vi "Update Chnls SyncHW.vi"(8 "error in (no error)":errorcluster, 10 "ChnlSettings":T1[](array[typedef]) {"ChnParameter"."Delay (µs)" min=0.0 max=100000000.0 format="%.4f"; "G08_Chnl_Settings"."Pulse Width (µs)" min=0.0 max=8947840.0 format="%#.6f"; "Go and Done Signal"."Done Signal" format="%04x" items=["Local Primary"=1, "Local Secondary"=2, "Local Force"=4, "Master Primary"=16]; "Go and Done Signal"."Go Signal" format="%04x" items=["Local Primary0x1"=1, "Local Secondary0x2"=2, "Local Force 0x4"=4, "Resynchronize 0x8"=8, "Master Prim. 0x10"=16, "Master Sec. 0x20"=32, "Master Force  0x40"=64, "System Clock 0x80"=128, "Delay Clock 0x100"=256, "Inhibit Local 0x200"=512, "Start Local 0x400"=1024, "Start Bus 0x800"=2048, "Step Back Local 0x1000"=4096, "Step Back Bus 0x2000"=8192, "RunCircle 0x4000"=16384, "SyncReload 0x8000"=32768, "From E 0x10000"=65536, "From F 0x20000"=131072, "From Bus 0x40000"=262144]}, 11 "BME_DG_System in":refnum<class "BME_DG_System.lvclass">) -> (0 "error out":errorcluster, 2 "ProblemChnls":string[](array[string]), 3 "BME_DG_System out":refnum<class "BME_DG_System.lvclass">)   [LabVIEW 2009, in "POLARIS BME DG.lvlib" / "BME_DG_System.lvclass"]
doc: "VI works with SG08P2 based systems. SG08P2 store new parameter in a buffer and waits for appropriate moment to activate they.\n\nFirst VI check the integrity of new chnl settints. Then it writes settings in channel objects. Last it uptates HW and call DLL SyncLoadAllCard. This allows the card to change to new parameters at next common output modulo counter. \n\n\n---------------\n\nauthor: Alexander Kessler, Helmholtz-Institut-Jena \nmaintainer: Alexander Kessler: alexander.kessler@uni-jena.de\n\n\nLicense Agreement for this software:\n\nCopyright (C)\nHelmholtz-Institut-Jena\nFröbelsteg 3\n07743 Jena\nGermany\n\nContact: alexander.kessler@uni-jena.de\n\nThis program is free software; you can redistribute it and/or modify it under the terms of the GNU General Public License as published by the Free Software Foundation; either version 2 of the license, or (at your option) any later version.\n\nThis program is distributed in the hope that it will be useful, but WITHOUT ANY WARRANTY; without even the implied warranty of MERCHANTABILITY or FITNESS FOR A PARTICULAR PURPOSE. See the GNU General License for more details (http://www.gnu.org)."
uses:
  BME_DG_System.lvclass
  LV-BME Interface/Chnl Settings Complete.ctl
  LV-BME Interface/ChnlSettings.ctl
  LV-BME Interface/Go_Done_Chnl_Settings.ctl
  LV-BME Interface/GoSignalBits.ctl
  LV-BME Interface/SG08_Chnl_Settings.ctl
  BME_DG_Chnl/BME_DG_Chnl.lvclass
  POLARIS BME DG.lvlib
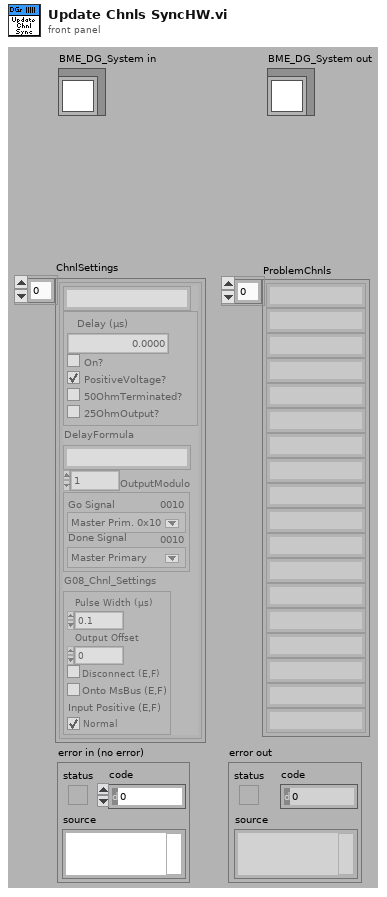
[diagram p1: front panel]
types:
  T1 = typedef "POLARIS BME DG.lvlib/Chnl Settings Complete.ctl" = cluster{"Channel Name":string, "ChnParameter":T2, "DelayFormula":string, "OutputModulo":i32, "Go and Done Signal":T3, "G08_Chnl_Settings":T5}
  T2 = typedef "POLARIS BME DG.lvlib/ChnlSettings.ctl" = cluster{" Delay (µs)":dbl, "On?":bool, "PositiveVoltage?":bool, "50OhmTerminated? ":bool, "25OhmOutput?":bool}
  T3 = typedef "POLARIS BME DG.lvlib/Go_Done_Chnl_Settings.ctl" = cluster{"Go Signal":T4, "Done Signal":u32}
  T4 = typedef "POLARIS BME DG.lvlib/GoSignalBits.ctl" = u32
  T5 = typedef "POLARIS BME DG.lvlib/SG08_Chnl_Settings.ctl" = cluster{"Pulse Width (µs)":dbl, "Output Offset":u32, "Disconnect (E,F)":bool, "Onto MsBus (E,F)":bool, "Input Positive (E,F)":bool}
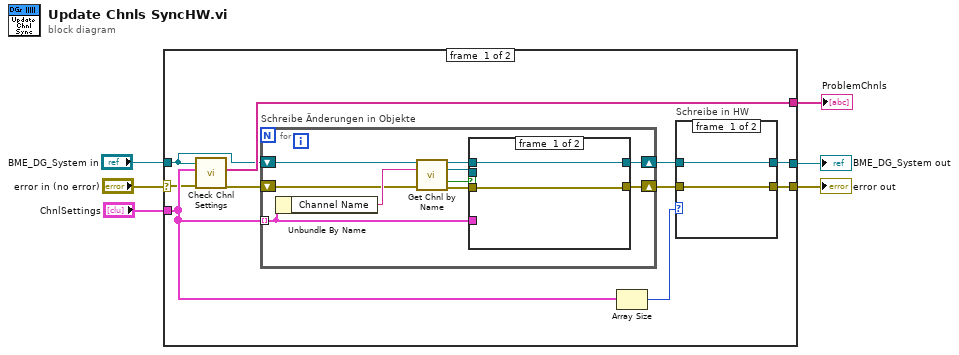
[diagram p0: block diagram]
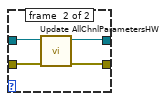
[diagram p2: hidden frame]
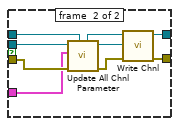
[diagram p3: hidden frame]
diagram:
  n1 = case shown="No Error" "error in (no error)" {
    selector: "error in (no error)" -> [w10 w45]
    tunnel: [w12 w45] -> w6
    tunnel: [w13 w44] -> w5
    tunnel: "BME_DG_System in" -> [w7 w44]
    tunnel: "ChnlSettings" -> [w11 _]
    tunnel: [w9 _] -> w1
    frame #0 {
      n2 = call "Check Chnl Settings.vi"("error in (no error)"=w10, "ChnlSettings"=w11, "BME_DG_System in"=w7) -> ("error out"=w8:errorcluster, "Problem Chnls out"=w9:string[])  [unwired: 7 in]
      n3 = for "Schreibe Änderungen in Objekte" {
        shift-right: [w27] -> w15
        shift-left: w7 -> [w28]
        tunnel: w11 -> [w23] mode=indexing
        shift-right: [w24] -> w14
        shift-left: w8 -> [w25]
        n4 = Unbundle By Name(w23) -> ("Channel Name"=w26:string)
        n5 = call "Get Chnl by Name.vi"("BME_DG_System in"=w28, "Chnl Name"=w26, "error in (no error)"=w25) -> ("BME_DG_System out"=w30:refnum<class "BME_DG_System.lvclass">, "BME_DG_Chnl"=w31:refnum<class "BME_DG_Chnl.lvclass">, "found?"=w32:bool, "error out"=w29:errorcluster)  [unwired: 7 in, 2 out]
        n6 = case shown="True" w32 {
          tunnel: w31 -> [_ w40]
          tunnel: w30 -> [w34 w38]
          tunnel: w29 -> [w33 w41]
          tunnel: [w34 w42] -> w27
          tunnel: [w33 w43] -> w24
          tunnel: w23 -> [_ w39]
          frame #0 {
          }
          frame #1 {
            n7 = call "Update All Chnl Parameter.vi"("BME_DG_System in"=w38, "error in (no error)"=w41, "ChnlSettings"=w39, "BME_DG_Chnl in"=w40) -> ("error out"=w36:errorcluster, "BME_DG_Chnl out"=w35:refnum<class "BME_DG_Chnl.lvclass">, "BME_DG_System out"=w37:refnum<class "BME_DG_System.lvclass">)  [unwired: 5 in]
            n8 = call "Write Chnl.vi"("error in (no error)"=w36, "BME_DG_Chnl.lvclass"=w35, "BME_DG_System in"=w37) -> ("error out"=w43:errorcluster, "BME_DG_System out"=w42:refnum<class "BME_DG_System.lvclass">)  [unwired: 7 in]
          }
        }
      }
      n9 = Array Size(array=w11) -> (size(s)=w16:i32)
      n10 = case "Schreibe in HW" shown="1, Default" w16 {
        tunnel: [w18 w20] -> w13
        tunnel: [w17 w19] -> w12
        tunnel: w15 -> [w18 w22]
        tunnel: w14 -> [w17 w21]
        frame #0 {
        }
        frame #1 {
          n11 = call "Update AllChnlParametersHW.vi"("error in (no error)"=w21, "BME_DG_System in"=w22) -> ("error out"=w19:errorcluster, "BME_DG_System out"=w20:refnum<class "BME_DG_System.lvclass">)  [unwired: 8 in]
        }
      }
    }
    frame #1 {
    }
  }
  "error out" <- w6
  "BME_DG_System out" <- w5
  "ProblemChnls" <- w1
